vi "myRIO_BRig_Host_endExp_main.vi"(11 "input_filePath":path) -> ()   [LabVIEW 2014]
panel:
  out "error out":errorcluster
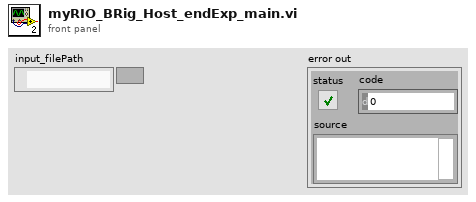
[diagram p1: front panel]
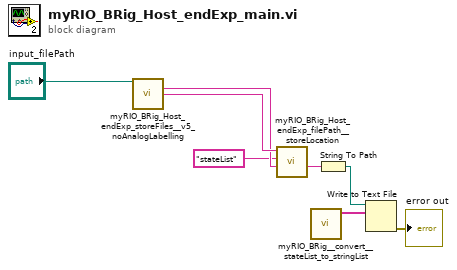
[diagram p0: block diagram]
diagram:
  n1 = call "myRIO_BRig_Host_endExp_storeFiles__v5_noAnalogLabelling.vi"("input_filePath"="input_filePath") -> ("output_expPrefix"=w6:string, "output_folderPath"=w7:string)  [unwired: 13 in]
  n2 = call "myRIO_BRig_Host_endExp_filePath__storeLocation.vi"("input_expPrefix"=w6, "input_fileName"="stateList", "input_filePath_storage"=w7) -> ("output_filePath"=w2:string)  [unwired: 8 in]
  n3 = call "myRIO_BRig__convert__stateList_to_stringList.vi"() -> ("Array"=w3:string[])  [unwired: 11 in]
  n4 = String To Path(string=w2) -> (path=w4:path)
  n5 = Write to Text File(file (use dialog)=w4, text=w3) -> (error out=→"error out":errorcluster)  [unwired: 2 in, 2 out]
